vi "NI VeriStand - Save Configuration File (Path).vi"(8 "Error in":errorcluster, 10 "File Path":string, 11 "Runtime Configuration Ref in":refnum<k24>) -> (0 "Error out":errorcluster, 2 "Success":bool, 3 "Runtime Configuration Ref out":refnum<k24>)   [LabVIEW 2025, in "NI_VS RuntimeConfigurationFile ScriptingAPI.lvlib"]
uses:
  NI_VS RuntimeConfigurationFile ScriptingAPI.lvlib
  NationalInstruments.VeriStand.SystemDefinitionAPI
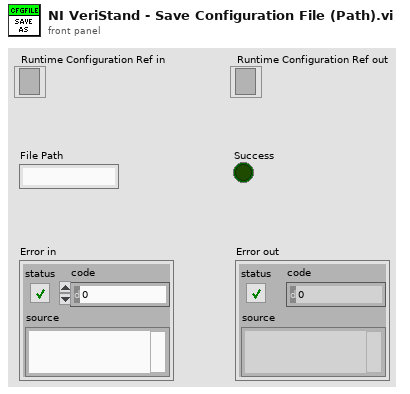
[diagram p1: front panel]
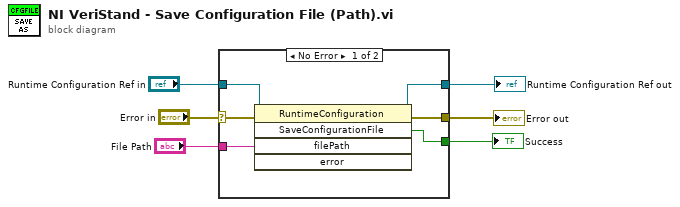
[diagram p0: block diagram]
diagram:
  n1 = case shown="No Error" "Error in" {
    selector: "Error in" -> [w11 _]
    tunnel: "Runtime Configuration Ref in" -> [w10 w13]
    tunnel: [w9 w13] -> w3
    tunnel: [w12 _] -> w6
    tunnel: "File Path" -> [w8 _]
    tunnel: [w7 _] -> w1
    frame No Error {
      n2 = invoke class="RuntimeConfiguration" method="SaveConfigurationFile"(reference=w10, error in=w11, "filePath"=w8) -> (reference out=w9:refnum<k24>, error out=w12:errorcluster, "SaveConfigurationFile"=w7:bool)  [unwired: 2 in, 2 out]
    }
    frame Error {
    }
  }
  "Runtime Configuration Ref out" <- w3
  "Success" <- w1
  "Error out" <- w6
